vi "Y Axis Scalar.vi"(11 "upper limit":dbl) -> (3 "Numeric":dbl)   [LabVIEW 2017]
uses:
  <vilib>/Rock Robotics/Network Tables/NT Read Number.vi
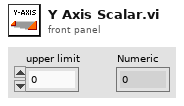
[diagram p1: front panel]
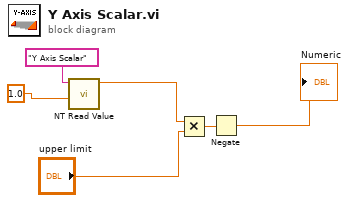
[diagram p0: block diagram]
diagram:
  n1 = call-poly <vilib>:"NT Read Value.vi"("Default Value"=1.0, "Name"="Y Axis Scalar") -> ("Numeric"=w3:dbl)  [unwired: 8 in, 1 out]
  n2 = Multiply(x=w3, y="upper limit") -> (x*y=w4:dbl)
  n3 = Negate(x=w4) -> (-x=→"Numeric":dbl)
